vi "IO_Sample.vi"   [LabVIEW 2014]
types:
  T1 = typedef "Data.ctl" = cluster{"Date":string, "BarCode1":string, "BarCode2":string, "BarCode3":string, "Message":string, "OK Count":u16, "NG Count":u16, "Total Count":u16, "ModelData":string[][], "OK&NG":bool, "COM1":refnum<visa-resource-name>, "COM2":refnum<visa-resource-name>, "IO":i32, "Time":u32, "TCP":refnum<k5>, "TCP 2":refnum<k5>, "COM3":refnum<visa-resource-name>}
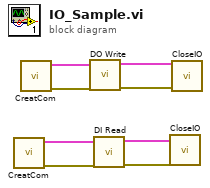
[diagram p0: block diagram]
diagram:
  n1 = call "CreatCom.vi"() -> ("error out"=w2:errorcluster, "Data Out"=w4:T1)  [unwired: 10 in]
  n2 = call "CreatCom.vi"() -> ("error out"=w7:errorcluster, "Data Out"=w8:T1)  [unwired: 10 in]
  n3 = call "DO Write.vi"("error in (no error)"=w7, "Data In"=w8) -> ("error out"=w5:errorcluster, "Data Out"=w6:T1)  [unwired: 8 in]
  n4 = call "DI Read.vi"("error in (no error)"=w2, "Data In"=w4) -> ("error out"=w1:errorcluster, "Data Out"=w3:T1)  [unwired: 7 in, 1 out]
  n5 = call "CloseIO.vi"("error in (no error)"=w1, "Data In"=w3) -> ()  [unwired: 8 in, 2 out]
  n6 = call "CloseIO.vi"("error in (no error)"=w5, "Data In"=w6) -> ()  [unwired: 8 in, 2 out]
